vi "AbortTest.vi"(8 "error in (no error)":errorcluster, 11 "reference in":refnum<class "Test_Template.lvclass">) -> (0 "error out":errorcluster, 3 "reference in":refnum<class "Test_Template.lvclass">)   [LabVIEW 2017]
uses:
  Test_Template.lvclass
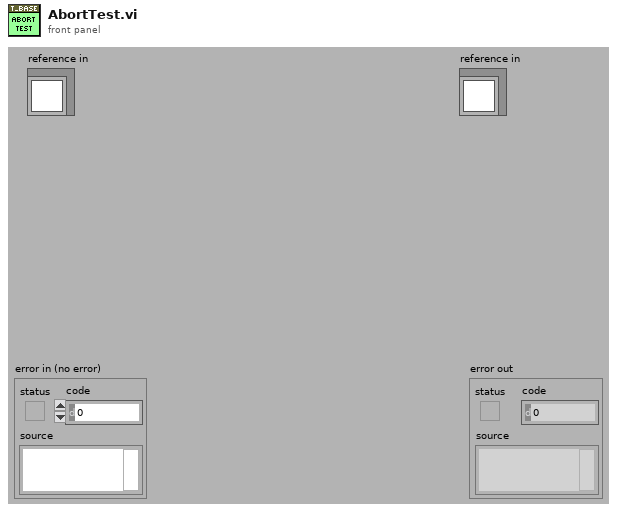
[diagram p1: front panel]
types:
  T1 = typedef "Test_Template.lvlib/Test_Template.lvclass/ObjectAttributes.ctl" = cluster{"Config":T2}
  T2 = typedef "Test_Template.lvlib/Test_Template.lvclass/Config.ctl" = cluster{"default":string}
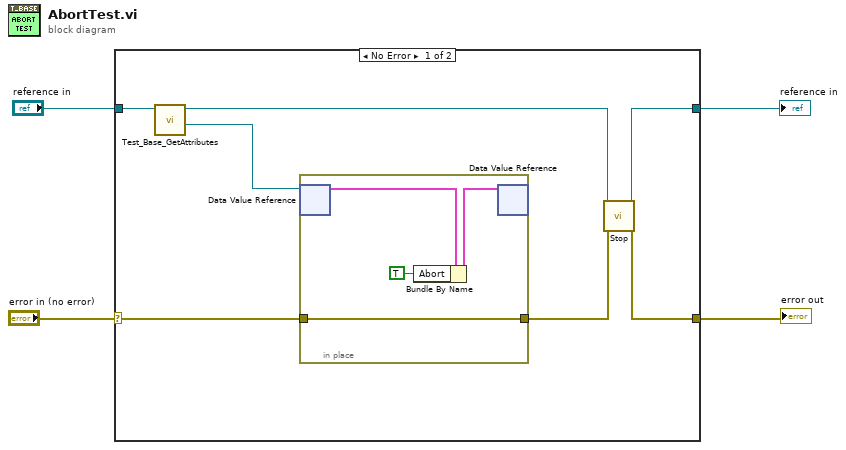
[diagram p0: block diagram]
diagram:
  n1 = case shown="No Error" "error in (no error)" {
    selector: "error in (no error)" -> [w6 w17]
    tunnel: [w5 w17] -> w3
    tunnel: [w8 w16] -> w1
    tunnel: "reference in" -> [w11 w16]
    frame No Error {
      n2 = call "Test_Base_GetAttributes.vi"("reference in"=w11) -> ("DataRef"=w10:refnum<data-value>, "reference out"=w9:refnum<class "Test_Template.lvclass">)  [unwired: 7 in, 2 out]
      n3 = in-place {
        in-place-border: [w12] -> w7
        in-place-border: w6 -> [w12]
        n4 = in-place-dvr #1(w10) -> (w15:T1)  [unwired: 1 out]
        n5 = Bundle By Name(cluster=w15, "Abort"=TRUE) -> (w14:T1)
        n6 = in-place-dvr #1(w14) -> ()  [unwired: 2 out]
      }
      n7 = call-dynamic "Stop.vi"("error in (no error)"=w7, "reference in"=w9) -> ("error out"=w5:errorcluster, "reference in"=w8:refnum<class "Test_Template.lvclass">)  [unwired: 8 in]
    }
    frame Error {
    }
  }
  "error out" <- w3
  "reference in" <- w1
